vi "VRM.Get Field.vi"(6 "Axis":T1=enum."Z", 8 "error in (no error)":errorcluster, 11 "Instrument.VRM in":refnum<class "Instrument.OxfordVRM.lvclass">) -> (0 "error out":errorcluster, 2 "Field (T)":dbl[](array[numeric]), 3 "Instrument.VRM out":refnum<class "Instrument.OxfordVRM.lvclass">)   [LabVIEW 2019, in "Instrument.OxfordVRM.lvclass"]
uses:
  Instrument.OxfordVRM.lvclass
  Typedefs/VRM Magnet Axis--Enum.ctl
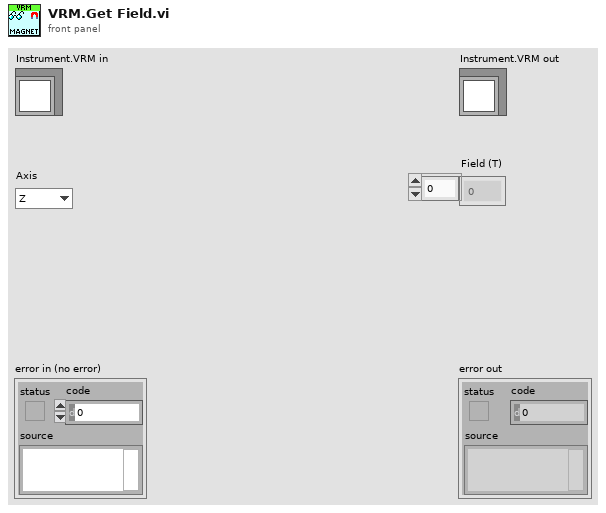
[diagram p1: front panel]
types:
  T1 = typedef "Instrument.OxfordVRM.lvclass/VRM Magnet Axis--Enum.ctl" = enum16{"X", "Y", "Z", "ALL"}
  T2 = typedef "Instrument.Cryostat.lvclass/Magnet Axis--Enum.ctl" = enum16{"X", "Y", "Z"}
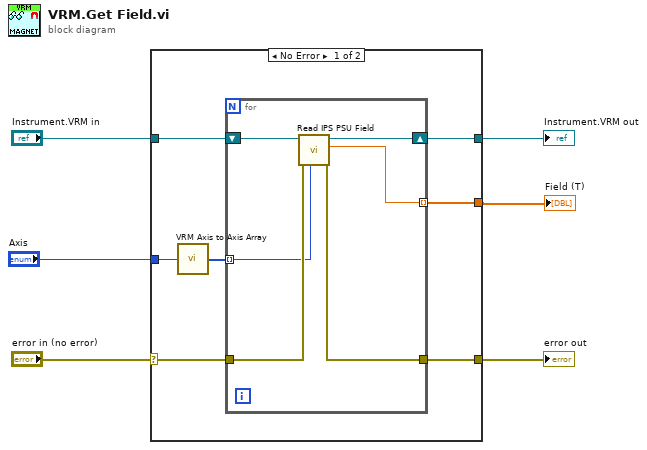
[diagram p0: block diagram]
diagram:
  n1 = case shown="No Error" "error in (no error)" {
    selector: "error in (no error)" -> [w11 w21]
    tunnel: [w10 w21] -> w3
    tunnel: [w12 w20] -> w1
    tunnel: "Instrument.VRM in" -> [w13 w20]
    tunnel: [w8 _] -> w2
    tunnel: "Axis" -> [w9 _]
    frame No Error {
      n2 = call "VRM Axis to Axis Array.vi"("Axis"=w9) -> ("Axis Array"=w7:T2[])
      n3 = for {
        tunnel: w7 -> [w15] mode=indexing
        tunnel: [w17] -> w8 mode=indexing
        shift-right: [w18] -> w12
        shift-left: w13 -> [w19]
        tunnel: w11 -> [w16]
        tunnel: [w14] -> w10
        n4 = call "Read IPS PSU Field.vi"("Axis"=w15, "error in (no error)"=w16, "Instrument.OxfordVRM in"=w19) -> ("error out"=w14:errorcluster, "Power Supply Field (T)"=w17:dbl, "Instrument.OxfordVRM out"=w18:refnum<class "Instrument.OxfordVRM.lvclass">)  [unwired: 6 in]
      }
    }
    frame Error {
    }
  }
  "error out" <- w3
  "Instrument.VRM out" <- w1
  "Field (T)" <- w2
